vi "RP EEprom to Voltage Scale.vi"(6 "EEPROM offset":i32=78, 9 "EEPROM range":u32=45870551, 10 "Signal bits":i32=14, 11 "Range":dbl=1.0 format="%#_6eV") -> (0 "Calibrated range":dbl, 1 "y intersept":dbl, 2 "Calibrated slope":dbl format="%#_27g", 3 "Slope":dbl)   [LabVIEW 2024]
panel:
  out "x << y":i32
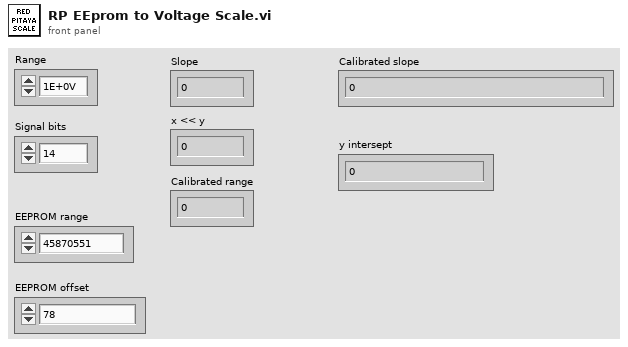
[diagram p1: front panel]
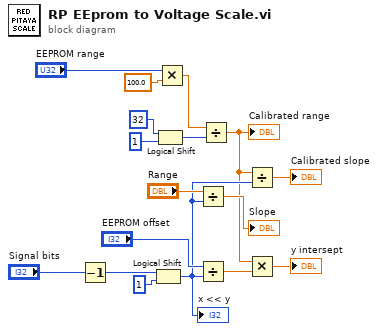
[diagram p0: block diagram]
diagram:
  n1 = Decrement(x="Signal bits") -> (x-1=w17:i32)
  n2 = Logical Shift(y=w17, x=1) -> (x << y=w3:i32)
  "x << y" <- w3
  n3 = Logical Shift(y=i16 32, x=u64 1) -> (x << y=w7:u64)
  n4 = Multiply(x="EEPROM range", y=100.0) -> (x*y=w8:dbl)
  n5 = Divide(x="Range", y=w3) -> (x/y=→"Slope":dbl)
  n6 = Divide(x="EEPROM offset", y=w3) -> (x/y=w5:dbl)
  n7 = Divide(x=w8, y=w7) -> (x/y=w1:dbl)
  "Calibrated range" <- w1
  n8 = Divide(x=w1, y=w3) -> (x/y=→"Calibrated slope":dbl)
  n9 = Multiply(x=w1, y=w5) -> (x*y=→"y intersept":dbl)
